vi "Resubscribe Following Reconnect.vi"(8 "error in":errorcluster, 10 "nats connection in":T1={"connection ID"=refnum, "server INFO"="", "timeout ms"=5000, "verbose?"=FALSE, "server headers?"=FALSE, "client headers?"=FALSE}, 11 "subs in":T2) -> (0 "error out":errorcluster)   [LabVIEW 2020, in "NATS Client.lvlib" / "NATS Client.lvclass"]
uses:
  NATS Client.lvclass
  NATS Subscription/NATS Subscription.lvclass
  NATS Subscription/NATS Subscription.lvclass/NATS Subscription.ctl
  <vilib>/NATS/NATS Core/NATS Core.lvlib
  Subscription Map.ctl
  <vilib>/NATS/NATS Core/Controls/nats connection.ctl
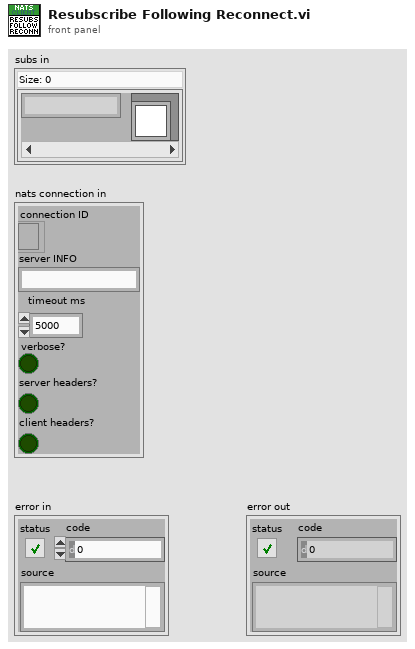
[diagram p1: front panel]
types:
  T1 = typedef "NATS Core.lvlib/nats connection.ctl" = cluster{"connection ID":refnum<k5>, "server INFO":string, "timeout ms":i32, "verbose?":bool, "server headers?":bool, "client headers?":bool}
  T2 = typedef "NATS Client.lvlib/NATS Client.lvclass/Subscription Map.ctl" = map{string, refnum<class "NATS Subscription.lvclass">}
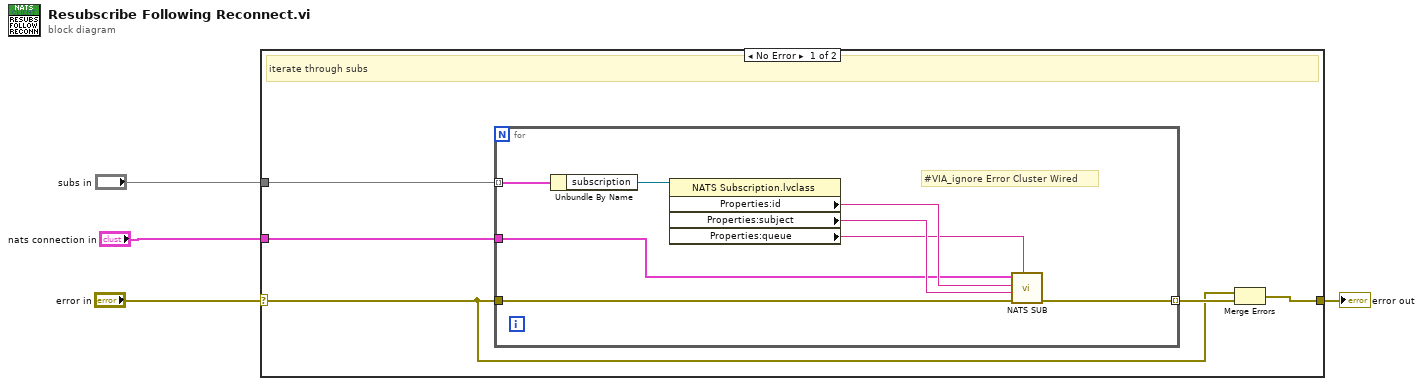
[diagram p0: block diagram]
diagram:
  n1 = case shown="No Error" "error in" {
    selector: "error in" -> [w5 w18]
    tunnel: "subs in" -> [w9 _]
    tunnel: [w6 w18] -> w1
    tunnel: "nats connection in" -> [w7 _]
    frame No Error {
      # "iterate through subs"
      n2 = for {
        tunnel: w9 -> [w17] mode=indexing
        tunnel: [w13] -> w8 mode=indexing
        tunnel: w5 -> [w12]
        tunnel: w7 -> [w11]
        # "#VIA_ignore Error Cluster Wired"
        n3 = Unbundle By Name(w17) -> ("subscription"=w16:refnum<class "NATS Subscription.lvclass">)
        n4 = property class="NATS Subscription.lvclass"(reference=w16) -> ("Properties:id"=w15:string, "Properties:subject"=w14:string, "Properties:queue"=w10:string)  [unwired: 1 in, 2 out]
        n5 = call <vilib>:"NATS SUB.vi"("queue group"=w10, "error in"=w12, "subject"=w14, "sub id"=w15, "nats connection in"=w11) -> ("error out"=w13:errorcluster)  [unwired: 4 in, 2 out]
      }
      n6 = Merge Errors(w5, w8) -> (w6:errorcluster)
    }
    frame Error {
    }
  }
  "error out" <- w1
